vi "array_to_xy-graph.vi"(1 "Input-Array":dbl[][](array[numeric]), 2 "y column":i32=2, 3 "x column":i32=1) -> (0 "graph":T1(graph))   [LabVIEW 2010]
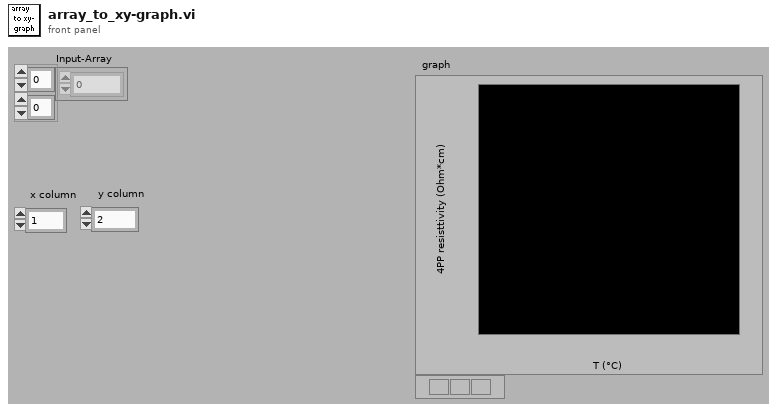
[diagram p1: front panel]
types:
  T1 = cluster{"Input-Array":dbl[], "Output-Array":dbl[]}
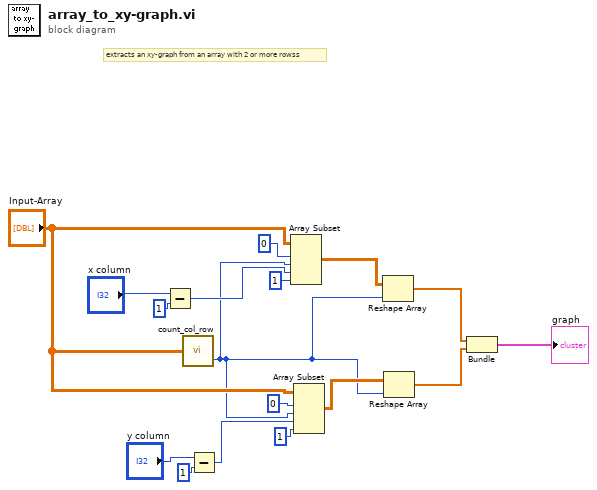
[diagram p0: block diagram]
diagram:
  # "extracts an xy-graph from an array with 2 or more rowss"
  n1 = Subtract(x="x column", y=1) -> (x-y=w8:i32)
  n2 = call "count_col_row.vi"("Input Array"="Input-Array") -> ("row"=w1:i32)  [unwired: 1 out]
  n3 = Subtract(x="y column", y=1) -> (x-y=w6:i32)
  n4 = Array Subset(array="Input-Array", index (row)=0 ("index"), length (row)=w1, index (col)=w8, length (col)=1 ("length")) -> (w4:dbl[][])
  n5 = Array Subset(array="Input-Array", index (row)=0 ("index"), length (row)=w1, index (col)=w6, length (col)=1 ("length")) -> (w3:dbl[][])
  n6 = Reshape Array(w4, w1) -> (w17:dbl[])
  n7 = Reshape Array(w3, w1) -> (w16:dbl[])
  n8 = Bundle "Bundle"(w17, w16) -> (→"graph":cluster{dbl[], dbl[]})  [unwired: 1 out]
